vi "libnodave_write_PLC.vi"(4 "inBuffer":u8[](array[numeric]), 5 "dataBlock":i32=-1, 6 "start":i32=-1, 7 "areaType":T1=132 items=["P Area"=128, "I Area"=129, "O Area"=130, "M Area"=131, "DB Area"=132, "Counter Area"=40, "Timer Area"=41], 8 "Error In":errorcluster, 9 "cpProtocol":i32=122, 10 "slot":i32=2, 11 "ip":string) -> (0 "Error Out":errorcluster, 2 "logInfo":string, 3 "return":i32)   [LabVIEW 2014]
doc: "This VI makes uses of the RADE_libnodave.dll, a C wrapper to the open-source libnodave library in order to write data to S-200, S-300 or S-400 PLCs. Recommend Caution while using this VI!"
uses:
  PLC_Libnodave_wrapper_areaType.ctl
  myDaveWrapper.dll
panel:
  # "RADE Libnodave PLC Write"
  # "RADE Libnodave PLC Write - Please use with Caution!"
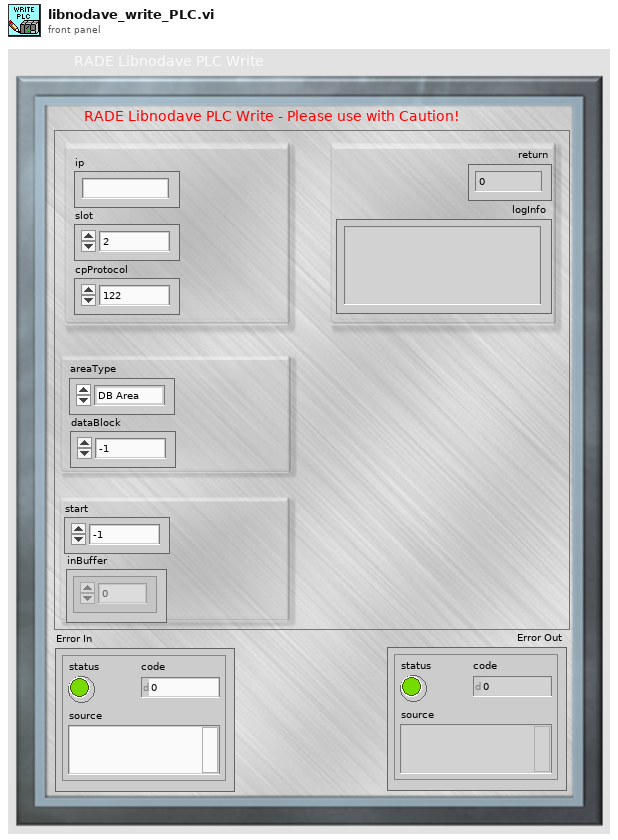
[diagram p1: front panel]
types:
  T1 = typedef "PLC_Libnodave_wrapper_areaType.ctl" = i32
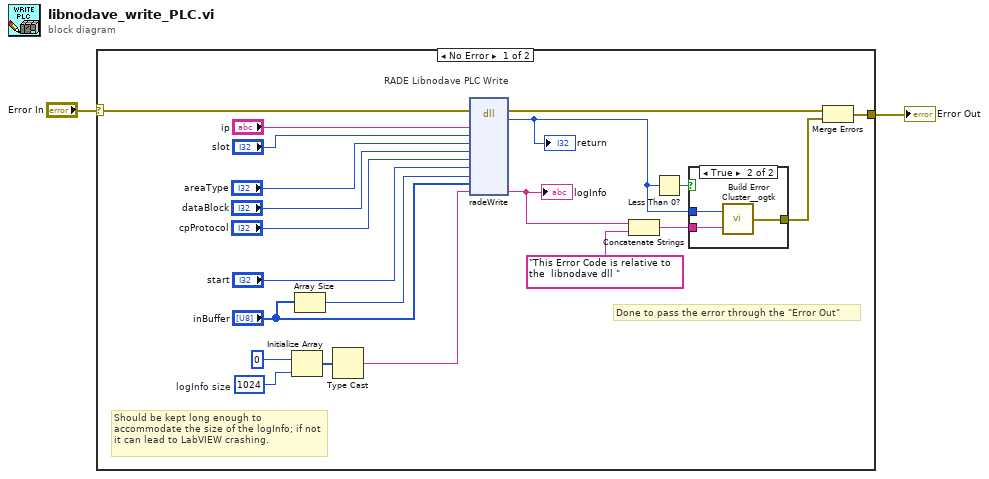
[diagram p0: block diagram]
diagram:
  n1 = case shown="No Error" "Error In" {
    selector: "Error In" -> [w11 w27]
    tunnel: [w5 w27] -> w1
    frame No Error {
      w18 = 1024  # logInfo size
      # "RADE Libnodave PLC Write"
      # "Done to pass the error through the \"Error Out\""
      # "Should be kept long enough to accommodate the size of the logInfo; if not it can lead to LabVIEW crashing."
      n2 = Initialize Array(u8 0, w18) -> (w16:u8[])
      n3 = Array Size(array="inBuffer") -> (size(s)=w14:i32)
      n4 = Type Cast(x=w16) -> (*(type *) &x=w15:string)  [unwired: 1 in]
      n5 = dll-call lib="C:/LabVIEW Projects/dave testing/Rade Wrapper/myDaveWrapper.dll" fn="radeWrite"(error in=w11, "ip"="ip", "slot"="slot", "areaType"="areaType", "dataBlock"="dataBlock", "cpProtocol"="cpProtocol", "start"="start", "length"=w14, "inBuffer"="inBuffer", "logInfo"=w15) -> (error out=w6:errorcluster, "return"=w9:i32, "logInfo"=w4:string)  [unwired: 10 in, 1 out]
      "return" <- w9
      "logInfo" <- w4
      n6 = Concatenate Strings(w4, "This Error Code is relative to the  libnodave dll " ("string")) -> (w3:string)
      n7 = Less Than 0?(x=w9) -> (x < 0?=w10:bool)
      n8 = case shown="True" w10 {
        tunnel: w3 -> [_ w26]
        tunnel: w9 -> [_ w25]
        tunnel: [_ w24] -> w7
        frame False {
        }
        frame True {
          n9 = call <userlib>:"Build Error Cluster__ogtk.vi"("String to Prepend to source (\"\")"=w26, "code"=w25) -> ("error out"=w24:errorcluster)
        }
      }
      n10 = Merge Errors(w6, w7) -> (w5:errorcluster)
    }
    frame Error {
    }
  }
  "Error Out" <- w1
